vi "tracking3.vi"(4 "lane keep":bool, 5 "reset path":bool, 6 "d":dbl=-0.1 format="%#_13g", 7 "car detection":bool, 8 "x3":dbl=15.0 format="%#_13g", 9 "x2":dbl=5.5 format="%#_13g", 10 "x1":dbl=5.0 format="%#_13g", 11 "xt":dbl) -> ()   [LabVIEW 2015]
uses:
  G_SEN.vi
  G_ALL.vi
  G_LCM.vi
panel:
  out "idx_start":i32
  out "lanedist":dbl
  out "idxx":dbl[](array[numeric])
  out "idx":dbl
  out "dist":dbl[](array[numeric])
  out "y origin":dbl[](array[numeric])
  out "x origin":dbl[](array[numeric])
  out "heading":dbl[](array[numeric])
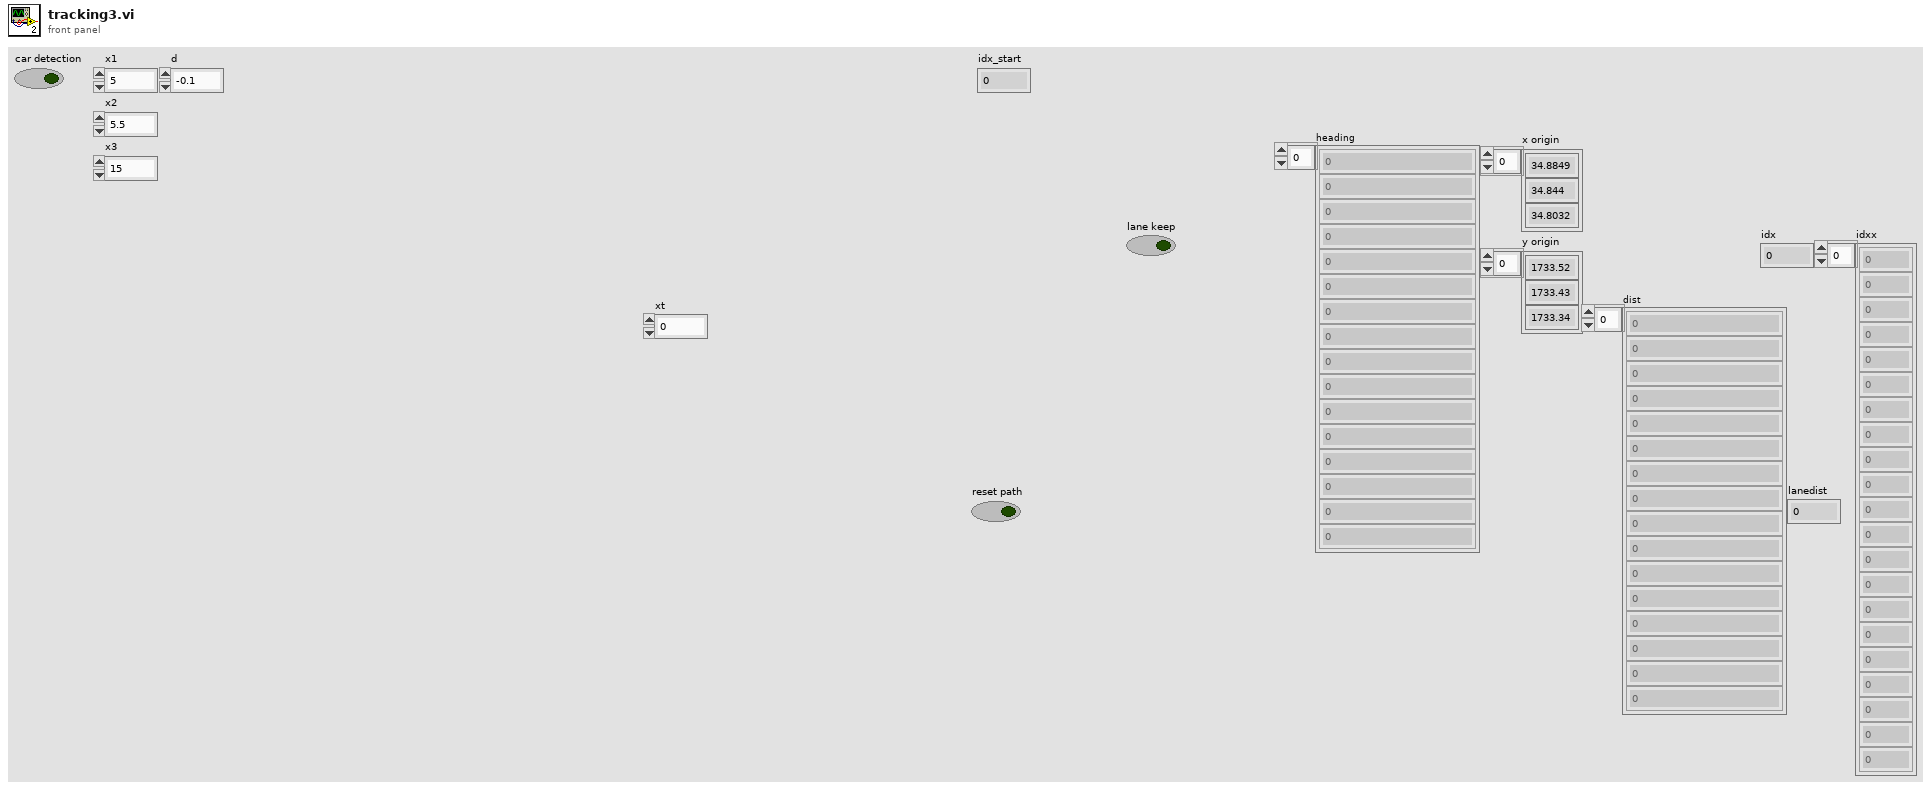
[diagram p1: front panel]
types:
  T1 = cluster{"Steer_input":dbl, "Steer_output":dbl, "VS_des":dbl, "VS_can":dbl, "heading":dbl, "auto":bool, "run":bool, "x":dbl, "y":dbl}
  T2 = cluster{"beep":bool, "duration (msec)":u32, "frequency (Hz)":u32}
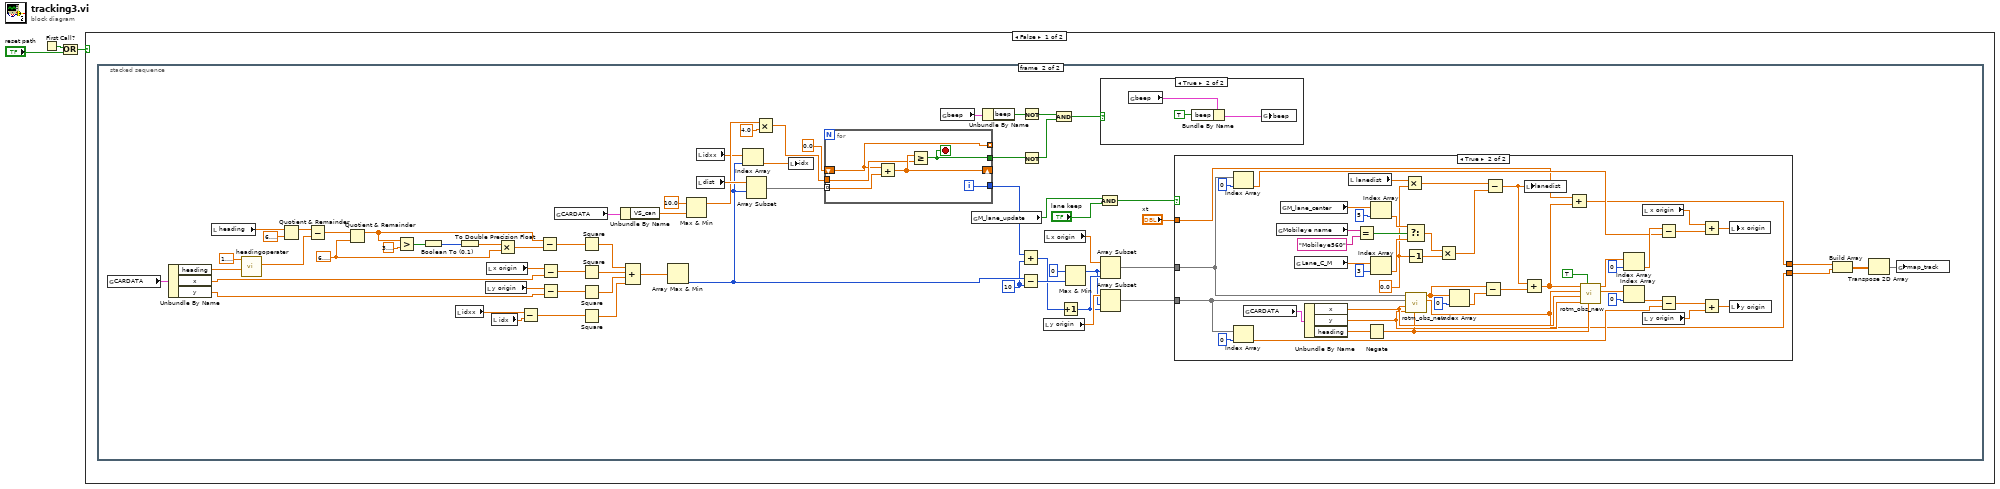
[diagram p0: block diagram]
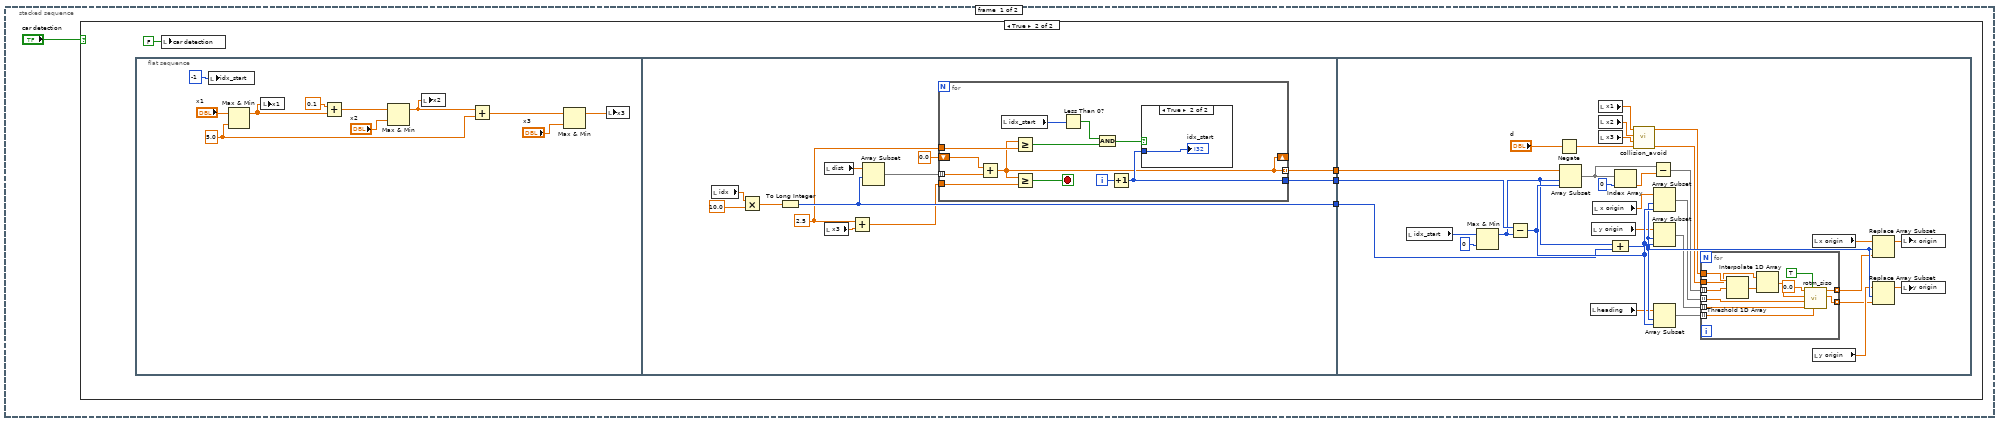
[diagram p2: hidden frame]
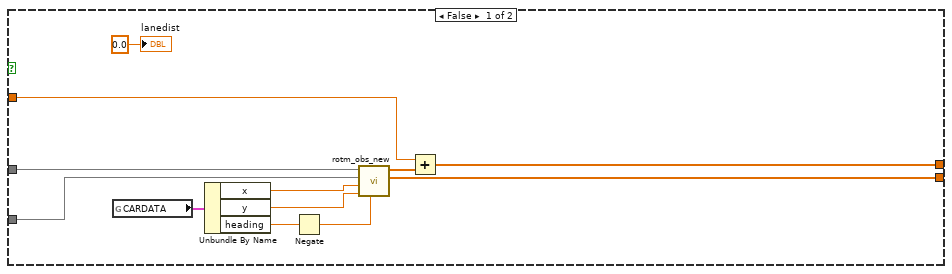
[diagram p6: hidden frame]
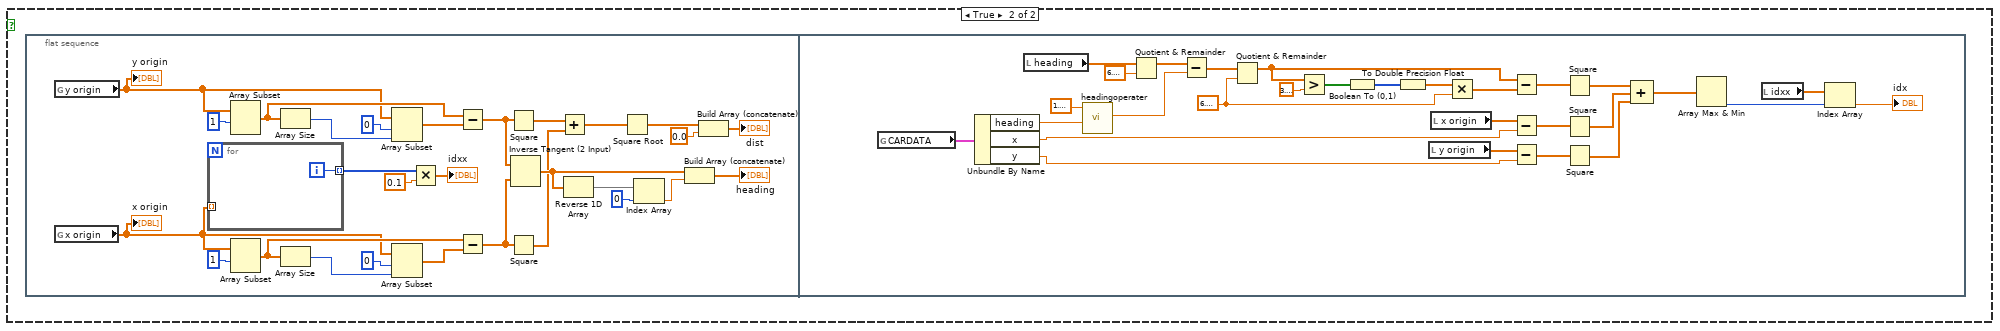
[diagram p7: hidden frame]
diagram:
  n1 = First Call?() -> (First Call?: T/F=w3:bool)
  n2 = Or(x=w3, y="reset path") -> (x .or. y?=w2:bool)
  n3 = case shown="False" w2 {
    frame False {
      n4 = stacked-sequence {
        frame #0 {
          n5 = case shown="True" "car detection" {
            frame False {
            }
            frame True {
              n6 = flat-sequence {
                tunnel: [w25] -> w7
                tunnel: [w24] -> w6
                tunnel: [w20] -> w5
                tunnel: w5 -> [w46]
                tunnel: w6 -> [w49]
                tunnel: w7 -> [w50]
                frame #0 {
                  w10 = 5.0 ("y")
                  n7 = local write "idx_start"(-1 ("idx_start")) -> ()
                  n8 = Max & Min(x="x1", y=w10) -> (max(x,y)=w16:dbl)  [unwired: 1 out]
                  n9 = local write "x1"(w16) -> ()
                  n10 = Add(x=0.1, y=w16) -> (x+y=w15:dbl)
                  n11 = Max & Min(x=w15, y="x2") -> (max(x,y)=w12:dbl)  [unwired: 1 out]
                  n12 = local write "x2"(w12) -> ()
                  n13 = Add(x=w12, y=w10) -> (x+y=w11:dbl)
                  n14 = Max & Min(x=w11, y="x3") -> (max(x,y)=w13:dbl)  [unwired: 1 out]
                  n15 = local write "x3"(w13) -> ()
                }
                frame #1 {
                  w21 = 2.5 ("y")
                  n16 = local read "idx"() -> (w31:dbl)
                  n17 = Multiply(x=w31, y=10.0) -> (x*y=w28:dbl)
                  n18 = To Long Integer(number=w28) -> (32bit integer=w25:i32)
                  n19 = local read "dist"() -> (w29:dbl[])
                  n20 = local read "x3"() -> (w23:dbl)
                  n21 = Add(x=w21, y=w23) -> (x+y=w22:dbl)
                  n22 = Array Subset(array=w29, index=w25) -> (w27:dbl[])  [unwired: 1 in]
                  n23 = for {
                    tunnel: w27 -> [w43] mode=indexing
                    shift-right: [w32] -> _
                    shift-left: 0.0 -> [w42]
                    tunnel: [w39] -> w24
                    tunnel: w22 -> [w38]
                    tunnel: w21 -> [w37]
                    tunnel: [w32] -> w20 mode=indexing
                    i -> [w40]
                    stop <- w41 stop-if-true
                    n24 = Add(x=w42, y=w43) -> (x+y=w32:dbl)
                    n25 = local read "idx_start"() -> (w36:i32)
                    n26 = Greater Or Equal?(x=w32, y=w37) -> (x >= y?=w33:bool)
                    n27 = Greater Or Equal?(x=w32, y=w38) -> (x >= y?=w41:bool)
                    n28 = Less Than 0?(x=w36) -> (x < 0?=w35:bool)
                    n29 = And(x=w35, y=w33) -> (x .and. y?=w34:bool)
                    n30 = Increment(x=w40) -> (x+1=w39:i32)
                    n31 = case shown="True" w34 {
                      tunnel: w39 -> [_ w44]
                      frame False {
                      }
                      frame True {
                        "idx_start" <- w44
                      }
                    }
                  }
                }
                frame #2 {
                  n32 = local read "idx_start"() -> (w48:i32)
                  n33 = Max & Min(x=w48, y=0) -> (max(x,y)=w45:i32)  [unwired: 1 out]
                  n34 = Subtract(x=w49, y=w45) -> (x-y=w74:i32)
                  n35 = Negate(x="d") -> (-x=w52:dbl)
                  n36 = Array Subset(array=w46, index=w45, length=w74) -> (w75:dbl[])
                  n37 = local read "heading"() -> (w58:dbl[])
                  n38 = local read "y origin"() -> (w67:dbl[])
                  n39 = local read "x origin"() -> (w72:dbl[])
                  n40 = local read "x1"() -> (w61:dbl)
                  n41 = local read "x2"() -> (w60:dbl)
                  n42 = local read "x3"() -> (w62:dbl)
                  n43 = Compound Arithmetic op=ADD(w45, w50) -> (w73:i32)
                  n44 = Index Array(array=w75, index=0) -> (element=w70:dbl)
                  n45 = call "collision_avoid.vi"("d"=w52, "x3"=w62, "x2"=w60, "x1"=w61) -> ("y"=w53:dbl[], "x"=w68:dbl[])  [unwired: 6 in]
                  n46 = Subtract(x=w75, y=w70) -> (x-y=w69:dbl[])
                  n47 = Array Subset(array=w72, index=w73, length=w74) -> (w59:dbl[])
                  n48 = Array Subset(array=w67, index=w73, length=w74) -> (w57:dbl[])
                  n49 = Array Subset(array=w58, index=w73, length=w74) -> (w56:dbl[])
                  n50 = for {
                    tunnel: w69 -> [w86] mode=indexing
                    tunnel: w68 -> [w87]
                    tunnel: w53 -> [w85]
                    tunnel: w59 -> [w83] mode=indexing
                    tunnel: w57 -> [w82] mode=indexing
                    tunnel: w56 -> [w81] mode=indexing
                    tunnel: [w80] -> w55 mode=indexing
                    tunnel: [w79] -> w54 mode=indexing
                    n51 = Threshold 1D Array(2:w86, 3:w87) -> (0:w84:dbl)  [unwired: 1 in]
                    n52 = Interpolate 1D Array(1:w84, 2:w85) -> (0:w76:dbl)
                    n53 = call "rotm_siso.vi"("angle[rad]"=w81, "reverse"=TRUE, "y0"=w82, "x0"=w83, "y"=w76, "x"=0.0 ("y")) -> ("y'"=w79:dbl, "x'"=w80:dbl)  [unwired: 4 in]
                  }
                  n54 = local read "x origin"() -> (w66:dbl[])
                  n55 = local read "y origin"() -> (w63:dbl[])
                  n56 = Replace Array Subset(array=w66, new element=w55, index=w73) -> (w65:dbl[])
                  n57 = Replace Array Subset(array=w63, new element=w54, index=w73) -> (w64:dbl[])
                  n58 = local write "x origin"(w65) -> ()
                  n59 = local write "y origin"(w64) -> ()
                }
              }
              n60 = local write "car detection"(FALSE ("Boolean")) -> ()
            }
          }
        }
        frame #1 {
          w90 = 10 ("y")
          w139 = 6.283185307179586
          n61 = global read "G_ALL.vi" "CARDATA"() -> (w102:T1)
          n62 = Unbundle By Name(w102) -> ("heading"=w133:dbl, "x"=w154:dbl, "y"=w152:dbl)
          n63 = local read "heading"() -> (w144:dbl[])
          n64 = call "headingoperater.vi"("h1"=w133, "h2"=1.5707963267948966) -> ("h2-h1"=w130:dbl)  [unwired: 8 in, 1 out]
          n65 = Quotient & Remainder(x=w144, y=6.283185307179586) -> (x-y*floor(x/y)=w145:dbl[])  [unwired: 1 out]
          n66 = Subtract(x=w145, y=w130) -> (x-y=w146:dbl[])
          n67 = Quotient & Remainder(x=w146, y=w139) -> (x-y*floor(x/y)=w147:dbl[])  [unwired: 1 out]
          n68 = Greater?(x=w147, y=3.141592653589793) -> (0:w143:bool[])
          n69 = Boolean To (0,1)(Boolean=w143) -> (0, 1=w142:i16[])
          n70 = local read "idxx"() -> (w113:dbl[])
          n71 = To Double Precision Float(number=w142) -> (double precision float=w140:dbl[])
          n72 = local read "y origin"() -> (w151:dbl[])
          n73 = local read "x origin"() -> (w153:dbl[])
          n74 = local read "idx"() -> (w114:dbl)
          n75 = Multiply(x=w140, y=w139) -> (x*y=w141:dbl[])
          n76 = Subtract(x=w113, y=w114) -> (x-y=w112:dbl[])
          n77 = Subtract(x=w147, y=w141) -> (x-y=w138:dbl[])
          n78 = Subtract(x=w153, y=w154) -> (x-y=w136:dbl[])
          n79 = Subtract(x=w151, y=w152) -> (x-y=w137:dbl[])
          n80 = global read "G_ALL.vi" "CARDATA"() -> (w101:T1)
          n81 = Square(x=w138) -> (x^2=w135:dbl[])
          n82 = Square(x=w136) -> (x^2=w132:dbl[])
          n83 = Square(x=w137) -> (x^2=w131:dbl[])
          n84 = Square(x=w112) -> (x^2=w111:dbl[])
          n85 = Unbundle By Name(w101) -> ("VS_can"=w100:dbl)
          n86 = Compound Arithmetic op=ADD(w135, w132, w131, w111) -> (w134:dbl[])
          n87 = Array Max & Min(array=w134) -> (min index (indices)=w96:i32)  [unwired: 3 out]
          n88 = Max & Min(x=10.0, y=w100) -> (max(x,y)=w127:dbl)  [unwired: 1 out]
          n89 = local read "idxx"() -> (w110:dbl[])
          n90 = local read "dist"() -> (w129:dbl[])
          n91 = Index Array(array=w110, index=w96) -> (element=w109:dbl)
          n92 = Array Subset(array=w129, index=w96) -> (w125:dbl[])  [unwired: 1 in]
          n93 = Multiply(x=w127, y=4.0) -> (x*y=w124:dbl)
          n94 = local write "idx"(w109) -> ()
          n95 = for {
            tunnel: w125 -> [w223] mode=indexing
            tunnel: w124 -> [w221]
            shift-right: [w222] -> _
            shift-left: 0.0 -> [w219]
            tunnel: [w220] -> w92
            tunnel: [w219] -> _ mode=indexing
            tunnel: [w218] -> w103
            i -> [w220]
            stop <- w218 stop-if-true
            n96 = Add(x=w219, y=w223) -> (x+y=w222:dbl)
            n97 = Greater Or Equal?(x=w222, y=w221) -> (x >= y?=w218:bool)
          }
          n98 = global read "G_ALL.vi" "beep"() -> (w98:T2)
          n99 = global read "G_SEN.vi" "M_lane_update"() -> (w119:bool)
          n100 = Unbundle By Name(w98) -> ("beep"=w97:bool)
          n101 = Add(x=w92, y=w90) -> (x+y=w91:i32)
          n102 = Subtract(x=w96, y=w90) -> (x-y=w95:i32)
          n103 = Not(x=w97) -> (.not. x?=w89:bool)
          n104 = Not(x=w103) -> (.not. x?=w88:bool)
          n105 = local read "y origin"() -> (w120:dbl[])
          n106 = local read "x origin"() -> (w121:dbl[])
          n107 = And(x=w89, y=w88) -> (x .and. y?=w106:bool)
          n108 = Increment(x=w91) -> (x+1=w104:i32)
          n109 = Max & Min(x=0, y=w95) -> (max(x,y)=w94:i32)  [unwired: 1 out]
          n110 = And(x=w119, y="lane keep") -> (x .and. y?=w118:bool)
          n111 = case shown="True" w106 {
            frame False {
            }
            frame True {
              n112 = global read "G_ALL.vi" "beep"() -> (w157:T2)
              n113 = Bundle By Name(cluster=w157, "beep"=TRUE) -> (w156:T2)
              n114 = global write "G_ALL.vi" "beep"(w156) -> ()
            }
          }
          n115 = Array Subset(array=w121, index=w94, length=w104) -> (w122:dbl[])
          n116 = Array Subset(array=w120, index=w94, length=w104) -> (w105:dbl[])
          n117 = case shown="True" w118 {
            tunnel: w122 -> [w165 w196]
            tunnel: w105 -> [w164 w194]
            tunnel: [w162 w179] -> w115
            tunnel: [w163 w181] -> w116
            tunnel: "xt" -> [w160 w178]
            frame False {
              n118 = global read "G_ALL.vi" "CARDATA"() -> (w158:T1)
              n119 = Unbundle By Name(w158) -> ("x"=w168:dbl, "y"=w167:dbl, "heading"=w169:dbl)
              n120 = Negate(x=w169) -> (-x=w166:dbl)
              n121 = call "rotm_obs_new.vi"("angle[rad]"=w166, "y0"=w167, "x0"=w168, "y"=w164, "x"=w165) -> ("rot*(y-y0) 2"=w163:dbl[], "rot*(x-x0)"=w161:dbl[])  [unwired: 3 in, 2 out]
              n122 = Add(x=w160, y=w161) -> (x+y=w162:dbl[])
              "lanedist" <- 0.0
            }
            frame True {
              w176 = 0.0 ("x")
              n123 = Index Array(array=w196, index=0) -> (element=w192:dbl)
              n124 = Index Array(array=w194, index=0) -> (element=w188:dbl)
              n125 = global read "G_ALL.vi" "CARDATA"() -> (w170:T1)
              n126 = global read "G_LCM.vi" "Mobileye name"() -> (w209:string)
              n127 = global read "G_SEN.vi" "M_lane_center"() -> (w204:dbl[])
              n128 = global read "G_SEN.vi" "Lane_C_M"() -> (w211:dbl[])
              n129 = Unbundle By Name(w170) -> ("x"=w202:dbl, "y"=w201:dbl, "heading"=w217:dbl)
              n130 = local read "lanedist"() -> (w177:dbl)
              n131 = Equal?(x=w209, y="Mobileye560") -> (x = y?=w207:bool)
              n132 = Negate(x=w217) -> (-x=w200:dbl)
              n133 = Index Array(array=w204, index=5) -> (element=w203:dbl)
              n134 = Index Array(array=w211, index=3) -> (element=w206:dbl)
              n135 = Multiply(x=w177, y=w176) -> (x*y=w173:dbl)
              n136 = Select(t=w203, s=w207, f=w206) -> (s? t:f=w175:dbl)
              n137 = Decrement(x=w176) -> (x-1=w174:dbl)
              n138 = call "rotm_obs_new.vi"("angle[rad]"=w200, "y0"=w201, "x0"=w202, "y"=w194, "x"=w196) -> ("rot*(y-y0) 2"=w181:dbl[], "rot*(x-x0)"=w214:dbl[])  [unwired: 3 in, 2 out]
              n139 = Multiply(x=w175, y=w174) -> (x*y=w172:dbl)
              n140 = Index Array(array=w214, index=0) -> (element=w215:dbl)
              n141 = Subtract(x=w214, y=w215) -> (x-y=w213:dbl[])
              n142 = Subtract(x=w173, y=w172) -> (x-y=w171:dbl)
              n143 = Add(x=w171, y=w213) -> (x+y=w180:dbl[])
              n144 = local write "lanedist"(w171) -> ()
              n145 = Add(x=w178, y=w180) -> (x+y=w179:dbl[])
              n146 = call "rotm_obs_new.vi"("angle[rad]"=w200, "reverse"=TRUE, "y0"=w201, "x0"=w202, "y"=w181, "x"=w180) -> ("rot*(y-y0) 2"=w190:dbl[], "rot*(x-x0)"=w199:dbl[])  [unwired: 2 in, 2 out]
              n147 = Index Array(array=w199, index=0) -> (element=w193:dbl)
              n148 = Index Array(array=w190, index=0) -> (element=w189:dbl)
              n149 = local read "x origin"() -> (w186:dbl[])
              n150 = local read "y origin"() -> (w184:dbl[])
              n151 = Subtract(x=w193, y=w192) -> (x-y=w187:dbl)
              n152 = Subtract(x=w189, y=w188) -> (x-y=w185:dbl)
              n153 = Add(x=w186, y=w187) -> (x+y=w183:dbl[])
              n154 = Add(x=w185, y=w184) -> (x+y=w182:dbl[])
              n155 = local write "x origin"(w183) -> ()
              n156 = local write "y origin"(w182) -> ()
            }
          }
          n157 = Build Array(w115, w116) -> (w117:dbl[][])
          n158 = Transpose 2D Array(2D array=w117) -> (transposed array=w99:dbl[][])
          n159 = global write "G_ALL.vi" "map_track"(w99) -> ()
        }
      }
    }
    frame True {
      n160 = flat-sequence {
        frame #0 {
          n161 = global read "G_ALL.vi" "y origin"() -> (w224:dbl[])
          "y origin" <- w224
          n162 = global read "G_ALL.vi" "x origin"() -> (w225:dbl[])
          "x origin" <- w225
          n163 = for {
            tunnel: w225 -> [_] mode=indexing
            tunnel: [w252] -> w228 mode=indexing
            i -> [w252]
          }
          n164 = Array Subset(array=w224, index=1) -> (w246:dbl[])  [unwired: 1 in]
          n165 = Array Subset(array=w225, index=1) -> (w247:dbl[])  [unwired: 1 in]
          n166 = Array Size(array=w246) -> (size(s)=w243:i32)
          n167 = Array Size(array=w247) -> (size(s)=w250:i32)
          n168 = Array Subset(array=w224, index=0, length=w243) -> (w245:dbl[])
          n169 = Array Subset(array=w225, index=0, length=w250) -> (w248:dbl[])
          n170 = Multiply(x=w228, y=0.1) -> (x*y=→"idxx":dbl[])
          n171 = Subtract(x=w246, y=w245) -> (x-y=w236:dbl[])
          n172 = Subtract(x=w247, y=w248) -> (x-y=w235:dbl[])
          n173 = Square(x=w236) -> (x^2=w234:dbl[])
          n174 = Square(x=w235) -> (x^2=w233:dbl[])
          n175 = Inverse Tangent (2 Input)(1:w235, 2:w236) -> (0:w237:dbl[])
          n176 = Add(x=w234, y=w233) -> (x+y=w232:dbl[])
          n177 = Reverse 1D Array(array=w237) -> (reversed array=w241:dbl[])
          n178 = Square Root(x=w232) -> (sqrt(x)=w231:dbl[])
          n179 = Index Array(array=w241, index=0) -> (element=w239:dbl)
          n180 = Build Array (concatenate)(w237, w239) -> (→"heading":dbl[])
          n181 = Build Array (concatenate)(w231, 0.0) -> (→"dist":dbl[])
        }
        frame #1 {
          w266 = 6.283185307179586
          n182 = global read "G_ALL.vi" "CARDATA"() -> (w253:T1)
          n183 = Unbundle By Name(w253) -> ("heading"=w260:dbl, "x"=w281:dbl, "y"=w279:dbl)
          n184 = local read "heading"() -> (w271:dbl[])
          n185 = call "headingoperater.vi"("h1"=w260, "h2"=1.5707963267948966) -> ("h2-h1"=w257:dbl)  [unwired: 8 in, 1 out]
          n186 = Quotient & Remainder(x=w271, y=6.283185307179586) -> (x-y*floor(x/y)=w272:dbl[])  [unwired: 1 out]
          n187 = Subtract(x=w272, y=w257) -> (x-y=w273:dbl[])
          n188 = Quotient & Remainder(x=w273, y=w266) -> (x-y*floor(x/y)=w274:dbl[])  [unwired: 1 out]
          n189 = Greater?(x=w274, y=3.141592653589793) -> (0:w270:bool[])
          n190 = Boolean To (0,1)(Boolean=w270) -> (0, 1=w269:i16[])
          n191 = To Double Precision Float(number=w269) -> (double precision float=w267:dbl[])
          n192 = local read "y origin"() -> (w278:dbl[])
          n193 = local read "x origin"() -> (w280:dbl[])
          n194 = Multiply(x=w267, y=w266) -> (x*y=w268:dbl[])
          n195 = Subtract(x=w274, y=w268) -> (x-y=w265:dbl[])
          n196 = Subtract(x=w280, y=w281) -> (x-y=w263:dbl[])
          n197 = Subtract(x=w278, y=w279) -> (x-y=w264:dbl[])
          n198 = Square(x=w265) -> (x^2=w262:dbl[])
          n199 = Square(x=w263) -> (x^2=w259:dbl[])
          n200 = Square(x=w264) -> (x^2=w258:dbl[])
          n201 = Compound Arithmetic op=ADD(w262, w259, w258) -> (w261:dbl[])
          n202 = Array Max & Min(array=w261) -> (min index (indices)=w255:i32)  [unwired: 3 out]
          n203 = local read "idxx"() -> (w256:dbl[])
          n204 = Index Array(array=w256, index=w255) -> (element=→"idx":dbl)
        }
      }
    }
  }
